vi "Display User Text Message.vi"(6 "Enable Lower Message (T: Enable)":bool, 7 "Enable Upper Message (T: Enable)":bool, 8 "error in (no error)":errorcluster, 9 "Lower Message (\"Message\")":string, 10 "Upper Message (\"Default\")":string, 11 "VISA resource name":refnum<visa-resource-name>) -> (0 "error out":errorcluster, 3 "VISA resource name out":refnum<visa-resource-name>)   [LabVIEW 2009, in "Keithley DMM7510.lvlib"]
doc: "This VI defines the text (both Top line and Bottom Line ) that is displayed on the front-panel USER swipe screen."
uses:
  Keithley DMM7510.lvlib
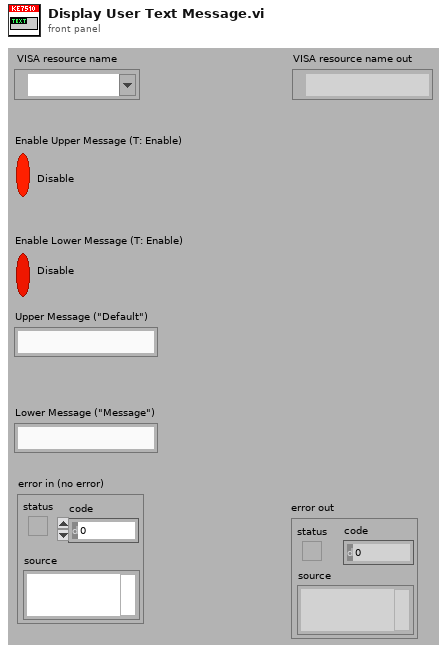
[diagram p1: front panel]
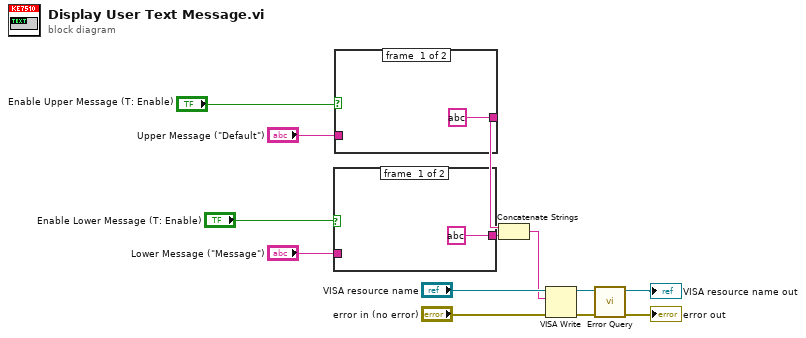
[diagram p0: block diagram]
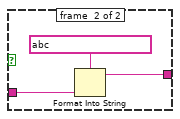
[diagram p2: hidden frame]
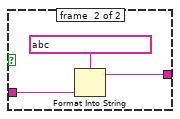
[diagram p3: hidden frame]
diagram:
  n1 = case shown="True" "Enable Lower Message (T: Enable)" {
    tunnel: [string ? w17] -> w3
    tunnel: "Lower Message (\"Message\")" -> [_ w15]
    frame #0 {
    }
    frame #1 {
      n2 = Format Into String(format string=string ?, w15) -> (resulting string=w17:string)  [unwired: 2 in, 1 out]
    }
  }
  n3 = case shown="True" "Enable Upper Message (T: Enable)" {
    tunnel: [string ? w21] -> w7
    tunnel: "Upper Message (\"Default\")" -> [_ w19]
    frame #0 {
    }
    frame #1 {
      n4 = Format Into String(format string=string ?, w19) -> (resulting string=w21:string)  [unwired: 2 in, 1 out]
    }
  }
  n5 = Concatenate Strings(w7, w3) -> (w4:string)
  n6 = VISA Write(VISA resource name="VISA resource name", write buffer=w4, error in (no error)="error in (no error)") -> (VISA resource name out=w11:refnum<visa-resource-name>, error out=w8:errorcluster)  [unwired: 1 out]
  n7 = call "Error Query.vi"("error in (no error)"=w8, "VISA resource name"=w11) -> ("error out"=→"error out":errorcluster, "VISA resource name out"=→"VISA resource name out":refnum<visa-resource-name>)  [unwired: 8 out]
